vi "Set Random Tracks.vi"(8 "error in (no error)":errorcluster, 10 "areas":i32, 11 "numTracks":i32) -> (0 "error out":errorcluster, 2 "areas out":i32, 3 "function return":u32)   [LabVIEW 2014, in "atmcd32d.lvlib"]
doc: "unsigned int WINAPI SetRandomTracks(int numTracks, int * areas);"
uses:
  atmcd32d.lvlib
  atmcd32d.dll
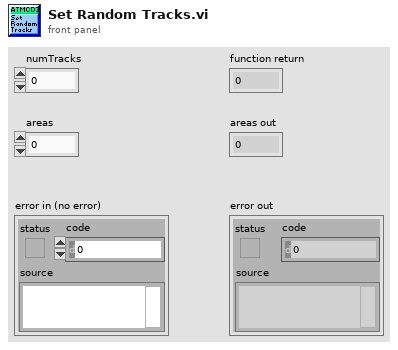
[diagram p1: front panel]
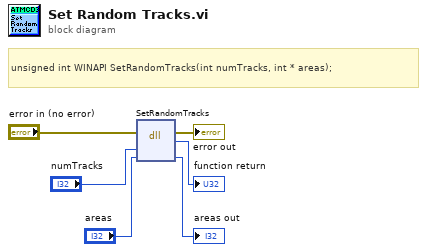
[diagram p0: block diagram]
diagram:
  # "unsigned int WINAPI SetRandomTracks(int numTracks, int * areas);"
  n1 = dll-call lib="C:/Users/Bakir/Documents/Lambda2-Testing/lib/Andorlib/atmcd32d.*" fn="SetRandomTracks"(error in="error in (no error)", "numTracks"="numTracks", "areas"="areas") -> (error out=→"error out":errorcluster, →"function return":u32, "areas"=→"areas out":i32)  [unwired: 3 in, 1 out]
